vi "input.vi"(8 "error in":errorcluster, 10 "data table in":T1, 11 "EthernetIP runtime in":refnum<class "EthernetIP runtime.lvclass">) -> (0 "error out":errorcluster, 2 "data table out":T1, 3 "EthernetIP runtime out":refnum<class "EthernetIP runtime.lvclass">)   [LabVIEW 2013, in "EthernetIP runtime.lvclass"]
doc: "Provides an interface for reading data from a module at runtime. While this interface performs no operations, a child should provide an override which may read from any open sessions, references, or interfaces."
uses:
  EthernetIP runtime.lvclass
  <vilib>/NI/Tag Bus/table/data table.ctl
  EthernetIP runtime.lvclass/EthernetIP runtime.ctl
  <vilib>/ethernetip/ethernetip.lvlib
  <vilib>/NI/Tag Bus/table/data table.lvlib
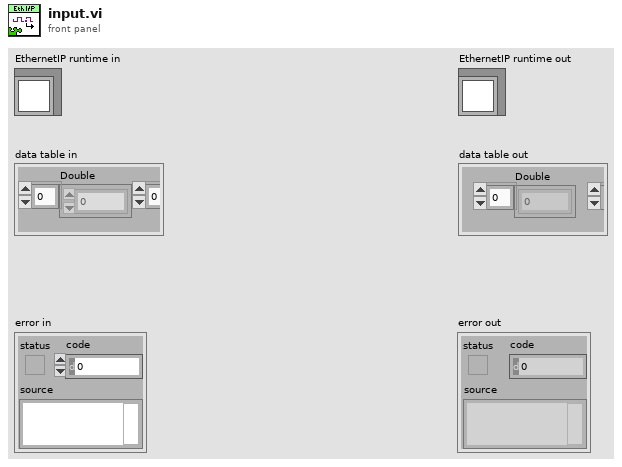
[diagram p1: front panel]
types:
  T1 = typedef "tag bus.lvlib/data table.lvlib/data table.ctl" = cluster{"Double":dbl[], "Single":sgl[], "I64":i64[], "I32":i32[], "I16":i16[], "I8":i8[], "U64":u64[], "U32":u32[], "U16":u16[], "U8":u8[], "Boolean":bool[], "String":string[], "Array of Double":cluster{"DBL Array":dbl[]}[], "Array of Single":cluster{"SGL Array":sgl[]}[], "Array of I64":cluster{"I64 Array":i64[]}[], "Array of I32":cluster{"I32 Array":i32[]}[], "Array of I16":cluster{"I16 Array":i16[]}[], "Array of I8":cluster{"I8 Array":i8[]}[], "Array of U64":cluster{"U64 Array":u64[]}[], "Array of U32":cluster{"U32 Array":u32[]}[], "Array of U16":cluster{"U16 Array":u16[]}[], "Array of U8":cluster{"U8 Array":u8[]}[], "Array of Boolean":cluster{"Boolean Array":bool[]}[], "Array of String":cluster{"String Array":string[]}[]}
  T2 = typedef "ethernetip.lvlib/ethernetip.ctl" = refnum<k21>
  T3 = typedef "EthernetIP runtime.lvclass/assembly data spec.ctl" = cluster{"Instance ID":u32, "specification":T4[]}
  T4 = typedef "EthernetIP runtime.lvclass/conversion specification.ctl" = cluster{"data type":T5, "data index":i32, "byte index":i32, "subindex":i32}
  T5 = typedef "tag bus.lvlib/tag descriptor.lvclass/Data Type.ctl" = enum16{"Double", "Single", "I64", "I32", "I16", "I8", "U64", "U32", "U16", "U8", "Boolean", "String", "Array of Double", "Array of Single", "Array of I64", "Array of I32", "Array of I16", "Array of I8", "Array of U64", "Array of U32", "Array of U16", "Array of U8", "Array of Boolean", "Array of String"}
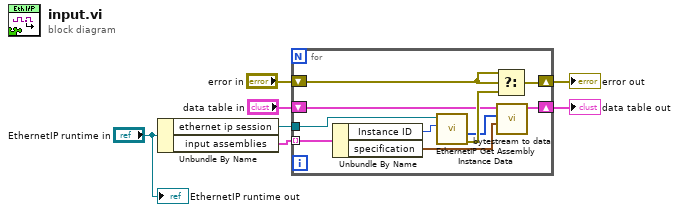
[diagram p0: block diagram]
diagram:
  n1 = Unbundle By Name("EthernetIP runtime in") -> ("ethernet ip session"=w6:T2, "input assemblies"=w3:T3[])
  n2 = for {
    tunnel: w6 -> [w17]
    shift-right: [w15] -> w4
    shift-left: "error in" -> [w16]
    tunnel: w3 -> [w13] mode=indexing
    shift-right: [w11] -> w1
    shift-left: "data table in" -> [w10]
    n3 = Unbundle By Name(w13) -> ("Instance ID"=w12:u32, "specification"=w8:T4[])
    n4 = call <vilib>:"EthernetIP Get Assembly Instance Data.vi"("Instance ID in"=w12, "Session in"=w17) -> ("error out"=w14:errorcluster, "Data"=w9:u8[])  [unwired: 6 in, 2 out]
    n5 = Select(t=w16, s=w16, f=w14) -> (s? t:f=w15:errorcluster)
    n6 = call "bytestream to data.vi"("specifications"=w8, "bytestream"=w9, "allocation"=w10) -> ("data table"=w11:T1)  [unwired: 8 in]
  }
  "error out" <- w4
  "data table out" <- w1
  "EthernetIP runtime out" <- "EthernetIP runtime in"
